vi "ex6-6.vi"   [LabVIEW 2013]
uses:
  <vilib>/NXT/Dual Mode Library/Sensors/EV3_Gyro_Angle.vi
  <vilib>/NXT/Dual Mode Library/Display/drawNumber_float.vi
  <vilib>/NXT/NXTIO Xnodes/NXTIONodeSubVIs/LEGOMoveAllMotors.vi
  <vilib>/NXT/Subs/LVHSConnector.ctl
  <vilib>/NXT/NXTIO Xnodes/NXTIOXNode/NXTIO.xnode
  <vilib>/NXT/LegoClasses/BrickReference/BrickReference.lvclass
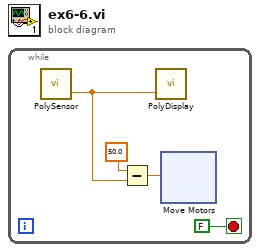
[diagram p0: block diagram]
diagram:
  n1 = while {
    stop <- FALSE stop-if-true
    n2 = call-poly <vilib>:"PolySensor.vi"() -> ("Degrees"=w1:sgl)  [unwired: 3 in, 1 out]
    n3 = Subtract(x=sgl 50.0, y=w1) -> (x-y=w3:sgl)
    n4 = call-poly <vilib>:"PolyDisplay.vi"("number"=w1) -> ()  [unwired: 3 in, 1 out]
    n5 = xnode "Move Motors"("Power/Speed 1"=w3) -> ()  [unwired: 2 in, 1 out]
  }
